vi "Ustawienie startu względem punktu o znanych współrzędnych.vi"(7 "Parametry odwzorowania\n Ziemi (WGS84)":cluster{"a":dbl, "b":dbl}, 8 "Punkt o znanych współrzędnych (baza)":T1, 10 "Ost. zazn. punkt [px]":T3) -> (3 "Poł. startu. out":T2)   [LabVIEW 2015, in "Biblioteka moduł map v3.lvlib" / "Pomocnicze.lvlib"]
uses:
  Pomocnicze/Pomocnicze.lvlib
  <vilib>/Utility/miscctls.llb/LVPoint32TypeDef.ctl
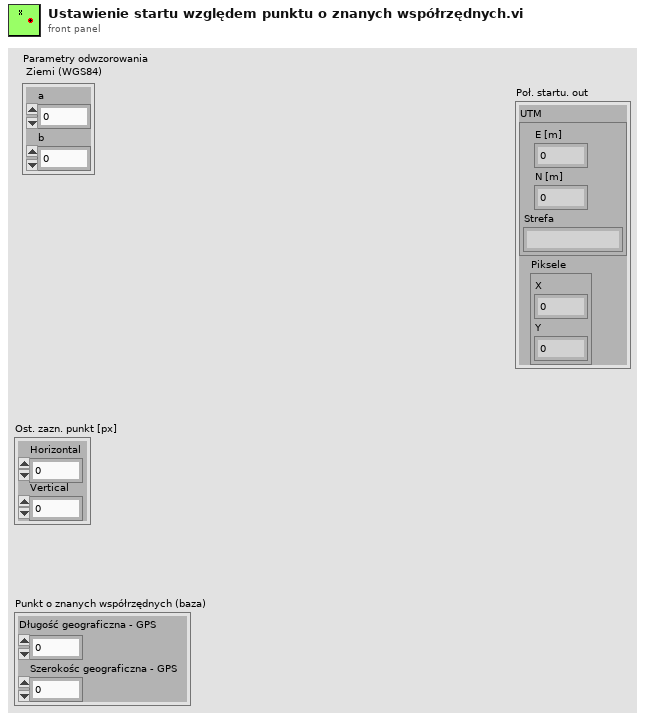
[diagram p1: front panel]
types:
  T1 = cluster{"Długość geograficzna - GPS":dbl, "Szerokośc geograficzna - GPS":dbl}
  T2 = cluster{"UTM":cluster{"E [m]":dbl, "N [m]":dbl, "Strefa":string}, "Piksele":cluster{"X":i32, "Y":i32}}
  T3 = typedef "LVPoint32TypeDef.ctl" = cluster{"Horizontal":i32, "Vertical":i32}
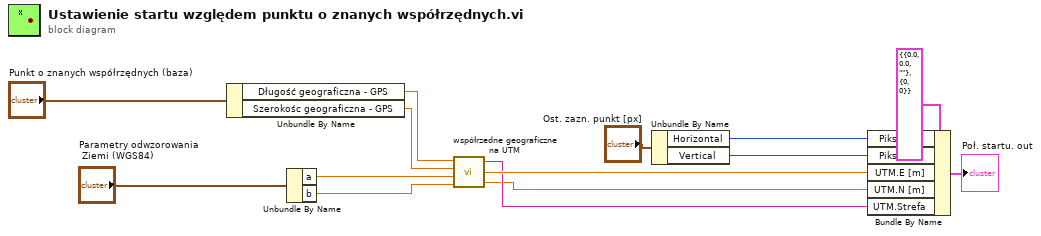
[diagram p0: block diagram]
diagram:
  n1 = Unbundle By Name("Punkt o znanych współrzędnych (baza)") -> ("Długość geograficzna - GPS"=w7:dbl, "Szerokośc geograficzna - GPS"=w8:dbl)
  n2 = Unbundle By Name("Parametry odwzorowania\n Ziemi (WGS84)") -> ("a"=w9:dbl, "b"=w10:dbl)
  n3 = call "współrzedne geograficzne na UTM.vi"("Położenie robota - długość geograficzna"=w7, "Położenie robota - szerokość geograficzna"=w8, "a"=w9, "b"=w10) -> ("Strefa"=w12:string, "E"=w13:dbl, "N"=w3:dbl)  [unwired: 2 in]
  n4 = Unbundle By Name("Ost. zazn. punkt [px]") -> ("Horizontal"=w2:i32, "Vertical"=w1:i32)
  n5 = Bundle By Name(cluster=T2 {"UTM"={"E [m]"=0.0, "N [m]"=0.0, "Strefa"=""}, "Piksele"={"X"=0, "Y"=0}} ("Poł. startu."), "Piksele.X"=w2, "Piksele.Y"=w1, "UTM.E [m]"=w13, "UTM.N [m]"=w3, "UTM.Strefa"=w12) -> (→"Poł. startu. out":T2)
